vi "Action.vi"(8 "error in (no error)":errorcluster, 10 "Actor in":refnum<class "Tamagotchi Basic Actor.lvclass">, 11 "Feed Message in":refnum<class "Feed Message.lvclass">) -> (0 "error out":errorcluster, 2 "Actor out":refnum<class "Tamagotchi Basic Actor.lvclass">, 3 "Feed Message out":refnum<class "Feed Message.lvclass">)   [LabVIEW 2026, in "Feed Message.lvclass"]
uses:
  Feed Message.lvclass
  Tamagotchi Basic Actor/Tamagotchi Basic Actor.lvclass
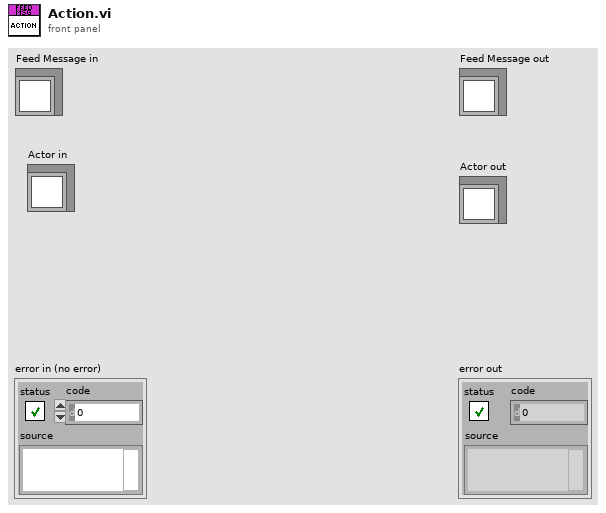
[diagram p1: front panel]
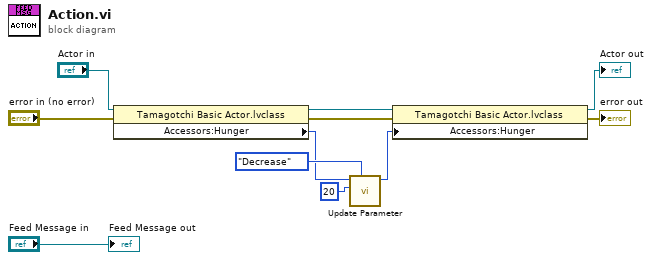
[diagram p0: block diagram]
diagram:
  n1 = property class="Tamagotchi Basic Actor.lvclass"(reference="Actor in", error in="error in (no error)") -> (reference out=w5:refnum<class "Tamagotchi Basic Actor.lvclass">, error out=w3:errorcluster, "Accessors:Hunger"=w8:i16)
  n2 = call "Update Parameter.vi"("Action"=enum16{"Increase", "Decrease"}."Decrease", "Modifier"=i16 20 ("y"), "Parameter"=w8) -> ("New Value"=w6:i16)  [unwired: 8 in]
  n3 = property class="Tamagotchi Basic Actor.lvclass"(reference=w5, error in=w3, "Accessors:Hunger"=w6) -> (reference out=→"Actor out":refnum<class "Tamagotchi Basic Actor.lvclass">, error out=→"error out":errorcluster)
  "Feed Message out" <- "Feed Message in"
